vi "Read Write Tests.vi"() -> ()   [LabVIEW 2021]
uses:
  <vilib>/Utility/Data Type/Type Definitions/Data Type.ctl
  <vilib>/TSA/Abstract Data Classes/Abs_Types/Type/Abs_Type.lvclass/Abs_Type.ctl
  Source/Omni-Bus/Omni_Bus.lvclass/Omni_Bus.ctl
  <vilib>/numeric/Random Number (Range) DBL.vi
  <vilib>/numeric/Random Number (Range) U64.vi
  <vilib>/numeric/Random Number (Range) I64.vi
  06a09804-3647-462b-9f8c-3b197f1d4842.vi
  d9e1931d-83c0-4008-a806-d0619767ccd4.vi
  22e3d29d-9de6-4bed-be07-da4388afe74d.vi
  4d5f569c-3ff8-4da6-911e-f6f6b6df5b4c.vi
  853aedcb-843d-4c1a-a070-a8abb42bd888.vi
  632325dd-8024-4226-85a2-78607102a822.vi
  31fcc082-04f4-426e-a822-d083f26efec9.vi
  a6d8fe4b-b8f8-4192-bfbd-ab0450d87a95.vi
  60e7b694-5e2b-40ae-be6d-936c5daed67f.vi
  0a5da363-2ab2-4b0a-bc23-95381a2f4f1f.vi
  f176570a-d467-4534-a5f4-80a5ed2f55fd.vi
  42086b41-aaa2-440a-9863-075bc68471ca.vi
  d6543037-67c4-4c9e-be04-516eba5ce324.vi
  8ee9f7fe-6a64-49fa-a0e4-dd7eef8eba2e.vi
  c8d26da6-dc4a-4689-8e38-86b886253208.vi
  282c234f-af01-4377-8eb2-d0f7920fef08.vi
  a689f72a-6438-4197-ae87-f9cf3b6f7a86.vi
  09187ef5-af96-4de4-9c12-a857a6033bec.vi
  d925c075-5a4f-45eb-b126-c84cbd9bef73.vi
  dbdc5551-9942-400f-9b9d-33a0d6ab74db.vi
  08a2d3fc-7221-4f6a-b613-8a00cd6bc1d4.vi
  211b282e-f175-4618-a45f-9254b3ae1368.vi
  ca77a7b4-ad37-4b73-9f94-404432450396.vi
  2a4b2bb2-c1db-44be-aa83-23dddfec57d5.vi
  b3c2ed11-8a20-4c33-b4f9-0e339c2323c2.vi
  ea50ac27-ce8e-4503-a9f0-9b9e5a91e659.vi
  6f7ce29f-c036-4842-ab22-8910a6a27a54.vi
  616da66d-3857-44c4-988f-95ea5e7f4ed6.vi
  b019b59e-0990-4c2e-a256-e10801dc45bc.vi
  c5feee88-916b-4341-8605-21dc42a231f5.vi
  3d3526cb-8a6e-48a6-bcab-e135716888a1.vi
  6cad3b51-a010-41ec-acd3-d4bb5fa17f8d.vi
  d0c0237e-e14a-450b-9942-79ec582db24b.vi
  ed5cb6ea-b411-43ee-bff1-ba243916202c.vi
  3a337c37-9261-480e-ae0e-8ba3684aa683.vi
  31c5e605-baef-4711-a879-1a5cd8a7ece4.vi
  4ecc3a5c-e12d-463c-8205-51799ca70095.vi
  330bfda6-5fcb-417b-a1fa-665fbbeb5077.vi
  9bcd3a16-7285-4366-9dfb-d430f520f572.vi
  <vilib>/numeric/sub_Random U32.vi
  Source/Omni-Bus/Write.vi
  Source/Omni-Bus/Support/Write/Write SGL.vi
  Source/Omni-Bus/Read.vi
  Source/Omni-Bus/Support/Read/Read SGL.vi
  Source/Omni-Bus/Support/Write/Write DBL.vi
  Source/Omni-Bus/Support/Read/Read DBL.vi
  Source/Omni-Bus/Support/Write/Write EXT.vi
  Source/Omni-Bus/Support/Read/Read EXT.vi
  Source/Omni-Bus/Support/Write/Write CSGL.vi
  Source/Omni-Bus/Support/Read/Read CSGL.vi
  Source/Omni-Bus/Support/Write/Write CDBL.vi
  Source/Omni-Bus/Support/Read/Read CDBL.vi
  Source/Omni-Bus/Support/Write/Write CEXT.vi
  Source/Omni-Bus/Support/Read/Read CEXT.vi
  Source/Omni-Bus/Support/Write/Write I8.vi
  Source/Omni-Bus/Support/Read/Read I8.vi
  Source/Omni-Bus/Support/Write/Write I16.vi
  Source/Omni-Bus/Support/Read/Read I16.vi
  Source/Omni-Bus/Support/Write/Write I32.vi
  Source/Omni-Bus/Support/Read/Read I32.vi
  Source/Omni-Bus/Support/Write/Write I64.vi
  Source/Omni-Bus/Support/Read/Read I64.vi
  Source/Omni-Bus/Support/Write/Write U8.vi
  Source/Omni-Bus/Support/Read/Read U8.vi
  Source/Omni-Bus/Support/Write/Write U16.vi
  Source/Omni-Bus/Support/Read/Read U16.vi
  Source/Omni-Bus/Support/Write/Write U32.vi
  Source/Omni-Bus/Support/Read/Read U32.vi
  Source/Omni-Bus/Support/Write/Write U64.vi
  Source/Omni-Bus/Support/Read/Read U64.vi
  Source/Omni-Bus/Support/Write/Write Time.vi
  Source/Omni-Bus/Support/Read/Read Time.vi
  Source/Omni-Bus/Support/Write/Write Boolean.vi
  Source/Omni-Bus/Support/Read/Read Boolean.vi
  Source/Omni-Bus/Support/Write/Write String.vi
  Source/Omni-Bus/Support/Read/Read String.vi
  Source/Omni-Bus/Support/Write/Write Variant.vi
  Source/Omni-Bus/Support/Read/Read Variant.vi
  Source/Omni-Bus/Support/Write/Write Waveform.vi
  Source/Omni-Bus/Support/Read/Read Waveform.vi
  Source/Omni-Bus/Support/Write/Write Multi SGL.vi
  Source/Omni-Bus/Support/Read/Read Multi SGL.vi
  Source/Omni-Bus/Support/Write/Write Multi DBL.vi
  Source/Omni-Bus/Support/Read/Read Multi DBL.vi
  Source/Omni-Bus/Support/Write/Write Multi EXT.vi
  Source/Omni-Bus/Support/Read/Read Multi EXT.vi
  Source/Omni-Bus/Support/Write/Write Multi CSGL.vi
  Source/Omni-Bus/Support/Read/Read Multi CSGL.vi
  Source/Omni-Bus/Support/Write/Write Multi CDBL.vi
  Source/Omni-Bus/Support/Read/Read Multi CDBL.vi
  Source/Omni-Bus/Support/Write/Write Multi CEXT.vi
  Source/Omni-Bus/Support/Read/Read Multi CEXT.vi
  Source/Omni-Bus/Support/Write/Write Multi I8.vi
  Source/Omni-Bus/Support/Read/Read Multi I8.vi
  Source/Omni-Bus/Support/Write/Write Multi I16.vi
  Source/Omni-Bus/Support/Read/Read Multi I16.vi
  Source/Omni-Bus/Support/Write/Write Multi I32.vi
  Source/Omni-Bus/Support/Read/Read Multi I32.vi
  Source/Omni-Bus/Support/Write/Write Multi I64.vi
  Source/Omni-Bus/Support/Read/Read Multi I64.vi
  Source/Omni-Bus/Support/Write/Write Multi U8.vi
  Source/Omni-Bus/Support/Read/Read Multi U8.vi
  Source/Omni-Bus/Support/Write/Write Multi U16.vi
  Source/Omni-Bus/Support/Read/Read Multi U16.vi
  Source/Omni-Bus/Support/Write/Write Multi U32.vi
  Source/Omni-Bus/Support/Read/Read Multi U32.vi
  Source/Omni-Bus/Support/Write/Write Multi U64.vi
  Source/Omni-Bus/Support/Read/Read Multi U64.vi
  Source/Omni-Bus/Support/Write/Write Multi Time.vi
  Source/Omni-Bus/Support/Read/Read Multi Time.vi
  Source/Omni-Bus/Support/Write/Write Multi Boolean.vi
  Source/Omni-Bus/Support/Read/Read Multi Boolean.vi
  Source/Omni-Bus/Support/Write/Write Multi String.vi
  Source/Omni-Bus/Support/Read/Read Multi String.vi
  Source/Omni-Bus/Support/Write/Write Multi Variant.vi
  Source/Omni-Bus/Support/Read/Read Multi Variant.vi
  Source/Omni-Bus/Support/Write/Write Multi Waveform.vi
  Source/Omni-Bus/Support/Read/Read Multi Waveform.vi
  Source/Omni-Bus/Support/FindVar.vi
  Source/Omni-Bus/Support/Get/Get Multi SGL.vi
  Source/Omni-Bus/Support/Get/Get Multi DBL.vi
  Source/Omni-Bus/Support/Get/Get Multi EXT.vi
  Source/Omni-Bus/Support/Get/Get Multi CPLX_SGL.vi
  Source/Omni-Bus/Support/Get/Get Multi CPLX_DBL.vi
  Source/Omni-Bus/Support/Get/Get Multi CPLX_EXT.vi
  Source/Omni-Bus/Support/Get/Get Multi I8.vi
  Source/Omni-Bus/Support/Get/Get Multi I16.vi
  Source/Omni-Bus/Support/Get/Get Multi I32.vi
  Source/Omni-Bus/Support/Get/Get Multi I64.vi
  Source/Omni-Bus/Support/Get/Get Multi U8.vi
  Source/Omni-Bus/Support/Get/Get Multi U16.vi
  Source/Omni-Bus/Support/Get/Get Multi U32.vi
  Source/Omni-Bus/Support/Get/Get Multi U64.vi
  Source/Omni-Bus/Support/Get/Get Multi Time.vi
  Source/Omni-Bus/Support/Get/Get Multi Boolean.vi
  Source/Omni-Bus/Support/Get/Get Multi String.vi
  Source/Omni-Bus/Support/Get/Get Multi Variant.vi
  Source/Omni-Bus/Support/Get/Get Multi Waveform.vi
  <vilib>/Utility/error.llb/Clear Errors.vi
  Source/Omni-Bus/Properties/Read Var Map.vi
  <vilib>/TSA/Abstract Data Classes/Abs_Types/Type/Properties/Read Tag.vi
  Source/Omni-Bus/Support/FindMultiVar.vi
  Source/Local Bus/Local Bus.lvclass
  C:/Users/Tim/Documents/GitHub/Omni-Bus/Source/Omni-Bus/Bus Access/Bus_Access.lvclass
  <vilib>/TSA/Abstract Data Classes/Abs_Types/Single Float/Abs_Single Float.lvclass
  C:/Program Files (x86)/National Instruments/LabVIEW 2021/vi.lib/TSA/Abstract Data Classes/Abs_Types/Type/Abs_Type.lvclass
  <vilib>/TSA/Abstract Data Classes/Abs_Types/Value/Abs_Value.lvclass
  <vilib>/TSA/Abstract Data Classes/Abs_Types/Double Float/Abs_Double Float.lvclass
  <vilib>/TSA/Abstract Data Classes/Abs_Types/Extended Float/Abs_Extended Float.lvclass
  <vilib>/TSA/Abstract Data Classes/Abs_Types/Complex Single Float/Abs_Complex Single Float.lvclass
  <vilib>/TSA/Abstract Data Classes/Abs_Types/Complex Double Float/Abs_Complex Double Float.lvclass
  <vilib>/TSA/Abstract Data Classes/Abs_Types/Complex Extended Float/Abs_Complex Extended Float.lvclass
  <vilib>/TSA/Abstract Data Classes/Abs_Types/I8 Integer/Abs_I8 Integer.lvclass
  <vilib>/TSA/Abstract Data Classes/Abs_Types/I16 Integer/Abs_I16 Integer.lvclass
  <vilib>/TSA/Abstract Data Classes/Abs_Types/I32 Integer/Abs_I32 Integer.lvclass
  <vilib>/TSA/Abstract Data Classes/Abs_Types/I64 Integer/Abs_I64 Integer.lvclass
  <vilib>/TSA/Abstract Data Classes/Abs_Types/U8 Integer/Abs_U8 Integer.lvclass
  <vilib>/TSA/Abstract Data Classes/Abs_Types/U16 Integer/Abs_U16 Integer.lvclass
  <vilib>/TSA/Abstract Data Classes/Abs_Types/U32 Integer/Abs_U32 Integer.lvclass
  <vilib>/TSA/Abstract Data Classes/Abs_Types/U64 Integer/Abs_U64 Integer.lvclass
  <vilib>/TSA/Abstract Data Classes/Abs_Types/Time/Abs_Time.lvclass
  <vilib>/TSA/Abstract Data Classes/Abs_Types/Boolean/Abs_Boolean.lvclass
  <vilib>/TSA/Abstract Data Classes/Abs_Types/String/Abs_String.lvclass
  <vilib>/TSA/Abstract Data Classes/Abs_Types/Variant/Abs_Variant.lvclass
  <vilib>/TSA/Abstract Data Classes/Abs_Types/Waveform/Abs_Waveform.lvclass
  <vilib>/addons/_JKI Toolkits/Caraya/classes/Test/Define Test.vi
  Source/Local Bus/Initialise - From List.vi
  Source/Omni-Bus/Support/Check For Read Only Error.vi
  Source/Omni-Bus/Support/Incorrect Tag String Error.vi
  <vilib>/addons/_JKI Toolkits/Caraya/classes/Assert/Assert.vi
  <vilib>/addons/_JKI Toolkits/Caraya/classes/Assert/Assert Not Error.vi
  <vilib>/addons/_JKI Toolkits/Caraya/classes/Assert/Assert Equal Value_Variant.vi
  Source/Omni-Bus/Omni_Bus.lvclass
  <vilib>/TSA/Abstract Data Classes/Abs_Types/Type/Abs_Type.lvclass
  <vilib>/Utility/Data Type/NI_Data Type.lvlib
  <vilib>/measure/NI_MAPro.lvlib
  <vilib>/measure/NI_MABase.lvlib
panel:
  out "error out":errorcluster
  in  "error in (no error)":errorcluster
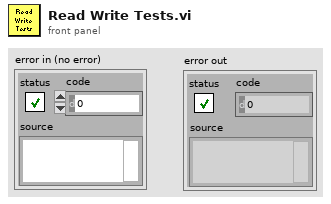
[diagram p1: front panel]
types:
  T1 = typedef "NI_Data Type.lvlib/Data Type.ctl" = enum8{"Invalid Type", "Void", "I8", "I16", "I32", "I64", "U8", "U16", "U32", "U64", "Single Float", "Double Float", "Extended Float", "Single Complex", "Double Complex", "Extended Complex", "Enum U8", "Enum U16", "Enum U32", "Enum U64", "Single Float With Unit", "Double Float With Unit", "Extended Float With Unit", "Single Complex with Unit", "Double Complex with Unit", "Extended Complex with Unit", "Boolean", "String", "Path", "Picture", "Tag", "Array", "Cluster", "Variant", "LV Variant", "Waveform", "Timestamp", "Digital Waveform", "Digital Data", "ExpressData", "Refnum", "External Data", "VI", "Poly VI", "LabVIEW Class Instance", "Fixed Point", "Set Collection", "Map Collection"}
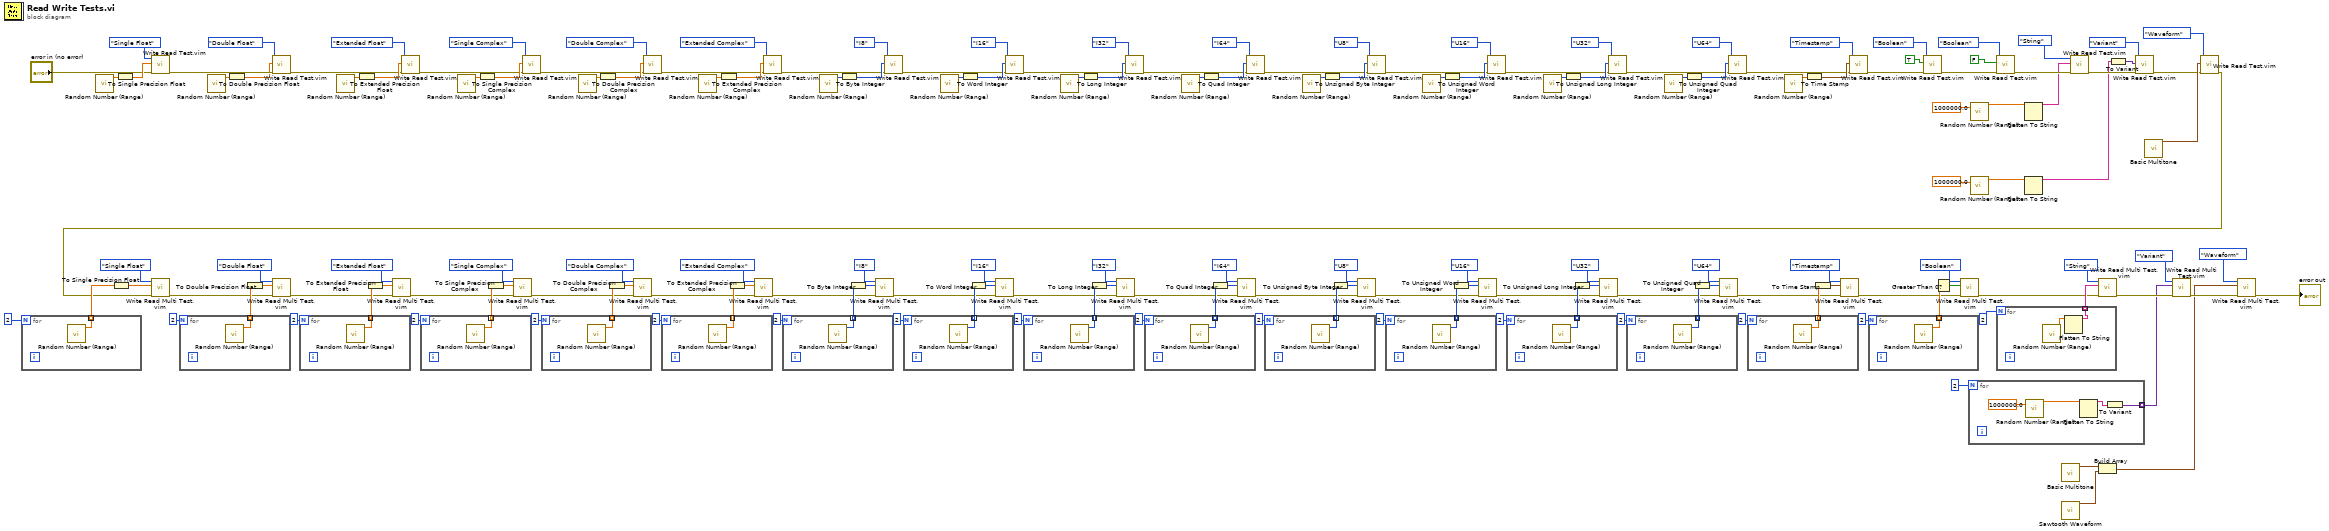
[diagram p0: block diagram]
diagram:
  n1 = for {
    N: 2 -> [_]
    tunnel: [w175] -> w92 mode=indexing
    n2 = call-poly <vilib>:"Random Number (Range).vi"() -> ("number"=w175:dbl)  [unwired: 11 in]
  }
  n3 = call-poly <vilib>:"Random Number (Range).vi"() -> ("number"=w171:dbl)  [unwired: 11 in]
  n4 = To Single Precision Float(number=w92) -> (single precision float=w91:sgl[])
  n5 = To Single Precision Float(number=w171) -> (single precision float=w170:sgl)
  n6 = call "Write Read Test.vim"("error in (no error)"="error in (no error)", "Test Value"=w170, "Type"=Data_Type."Single Float") -> ("error out"=w173:errorcluster)  [unwired: 8 in]
  n7 = for {
    N: 2 -> [_]
    tunnel: [w176] -> w88 mode=indexing
    n8 = call-poly <vilib>:"Random Number (Range).vi"() -> ("number"=w176:dbl)  [unwired: 11 in]
  }
  n9 = call-poly <vilib>:"Random Number (Range).vi"() -> ("number"=w169:dbl)  [unwired: 11 in]
  n10 = To Double Precision Float(number=w169) -> (double precision float=w168:dbl)
  n11 = To Double Precision Float(number=w88) -> (double precision float=w89:dbl[])
  n12 = call "Write Read Test.vim"("error in (no error)"=w173, "Test Value"=w168, "Type"=Data_Type."Double Float") -> ("error out"=w164:errorcluster)  [unwired: 8 in]
  n13 = for {
    N: 2 -> [_]
    tunnel: [w177] -> w82 mode=indexing
    n14 = call-poly <vilib>:"Random Number (Range).vi"() -> ("number"=w177:dbl)  [unwired: 11 in]
  }
  n15 = call-poly <vilib>:"Random Number (Range).vi"() -> ("number"=w166:dbl)  [unwired: 11 in]
  n16 = To Extended Precision Float(1:w166) -> (0:w167:ext)
  n17 = To Extended Precision Float(1:w82) -> (0:w81:ext[])
  n18 = call "Write Read Test.vim"("error in (no error)"=w164, "Test Value"=w167, "Type"=Data_Type."Extended Float") -> ("error out"=w160:errorcluster)  [unwired: 8 in]
  n19 = for {
    N: 2 -> [_]
    tunnel: [w178] -> w79 mode=indexing
    n20 = call-poly <vilib>:"Random Number (Range).vi"() -> ("number"=w178:dbl)  [unwired: 11 in]
  }
  n21 = call-poly <vilib>:"Random Number (Range).vi"() -> ("number"=w162:dbl)  [unwired: 11 in]
  n22 = To Single Precision Complex(1:w162) -> (0:w161:csg)
  n23 = To Single Precision Complex(1:w79) -> (0:w80:csg[])
  n24 = call "Write Read Test.vim"("error in (no error)"=w160, "Test Value"=w161, "Type"=Data_Type."Single Complex") -> ("error out"=w156:errorcluster)  [unwired: 8 in]
  n25 = for {
    N: 2 -> [_]
    tunnel: [w179] -> w74 mode=indexing
    n26 = call-poly <vilib>:"Random Number (Range).vi"() -> ("number"=w179:dbl)  [unwired: 11 in]
  }
  n27 = call-poly <vilib>:"Random Number (Range).vi"() -> ("number"=w158:dbl)  [unwired: 11 in]
  n28 = To Double Precision Complex(1:w158) -> (0:w159:cdb)
  n29 = To Double Precision Complex(1:w74) -> (0:w73:cdb[])
  n30 = call "Write Read Test.vim"("error in (no error)"=w156, "Test Value"=w159, "Type"=Data_Type."Double Complex") -> ("error out"=w152:errorcluster)  [unwired: 8 in]
  n31 = for {
    N: 2 -> [_]
    tunnel: [w180] -> w71 mode=indexing
    n32 = call-poly <vilib>:"Random Number (Range).vi"() -> ("number"=w180:dbl)  [unwired: 11 in]
  }
  n33 = call-poly <vilib>:"Random Number (Range).vi"() -> ("number"=w154:dbl)  [unwired: 11 in]
  n34 = To Extended Precision Complex(1:w154) -> (0:w153:cxt)
  n35 = To Extended Precision Complex(1:w71) -> (0:w72:cxt[])
  n36 = call "Write Read Test.vim"("error in (no error)"=w152, "Test Value"=w153, "Type"=Data_Type."Extended Complex") -> ("error out"=w148:errorcluster)  [unwired: 8 in]
  n37 = for {
    N: 2 -> [_]
    tunnel: [w181] -> w66 mode=indexing
    n38 = call-poly <vilib>:"Random Number (Range).vi"() -> ("number"=w181:i64)  [unwired: 11 in]
  }
  n39 = call-poly <vilib>:"Random Number (Range).vi"() -> ("number"=w150:i64)  [unwired: 11 in]
  n40 = To Byte Integer(number=w150) -> (8bit integer=w151:i8)
  n41 = To Byte Integer(number=w66) -> (8bit integer=w65:i8[])
  n42 = call "Write Read Test.vim"("error in (no error)"=w148, "Test Value"=w151, "Type"=Data_Type."I8") -> ("error out"=w144:errorcluster)  [unwired: 8 in]
  n43 = for {
    N: 2 -> [_]
    tunnel: [w182] -> w63 mode=indexing
    n44 = call-poly <vilib>:"Random Number (Range).vi"() -> ("number"=w182:i64)  [unwired: 11 in]
  }
  n45 = call-poly <vilib>:"Random Number (Range).vi"() -> ("number"=w146:i64)  [unwired: 11 in]
  n46 = To Word Integer(number=w146) -> (16bit integer=w145:i16)
  n47 = To Word Integer(number=w63) -> (16bit integer=w64:i16[])
  n48 = call "Write Read Test.vim"("error in (no error)"=w144, "Test Value"=w145, "Type"=Data_Type."I16") -> ("error out"=w140:errorcluster)  [unwired: 8 in]
  n49 = for {
    N: 2 -> [_]
    tunnel: [w183] -> w58 mode=indexing
    n50 = call-poly <vilib>:"Random Number (Range).vi"() -> ("number"=w183:i64)  [unwired: 11 in]
  }
  n51 = call-poly <vilib>:"Random Number (Range).vi"() -> ("number"=w142:i64)  [unwired: 11 in]
  n52 = To Long Integer(number=w142) -> (32bit integer=w143:i32)
  n53 = To Long Integer(number=w58) -> (32bit integer=w57:i32[])
  n54 = call "Write Read Test.vim"("error in (no error)"=w140, "Test Value"=w143, "Type"=Data_Type."I32") -> ("error out"=w136:errorcluster)  [unwired: 8 in]
  n55 = for {
    N: 2 -> [_]
    tunnel: [w184] -> w55 mode=indexing
    n56 = call-poly <vilib>:"Random Number (Range).vi"() -> ("number"=w184:i64)  [unwired: 11 in]
  }
  n57 = call-poly <vilib>:"Random Number (Range).vi"() -> ("number"=w138:i64)  [unwired: 11 in]
  n58 = To Quad Integer(1:w138) -> (0:w137:i64)
  n59 = To Quad Integer(1:w55) -> (0:w56:i64[])
  n60 = call "Write Read Test.vim"("error in (no error)"=w136, "Test Value"=w137, "Type"=Data_Type."I64") -> ("error out"=w132:errorcluster)  [unwired: 8 in]
  n61 = for {
    N: 2 -> [_]
    tunnel: [w185] -> w50 mode=indexing
    n62 = call-poly <vilib>:"Random Number (Range).vi"() -> ("number"=w185:u64)  [unwired: 11 in]
  }
  n63 = call-poly <vilib>:"Random Number (Range).vi"() -> ("number"=w134:u64)  [unwired: 11 in]
  n64 = To Unsigned Byte Integer(number=w134) -> (unsigned 8bit integer=w135:u8)
  n65 = To Unsigned Byte Integer(number=w50) -> (unsigned 8bit integer=w49:u8[])
  n66 = call "Write Read Test.vim"("error in (no error)"=w132, "Test Value"=w135, "Type"=Data_Type."U8") -> ("error out"=w128:errorcluster)  [unwired: 8 in]
  n67 = for {
    N: 2 -> [_]
    tunnel: [w186] -> w47 mode=indexing
    n68 = call-poly <vilib>:"Random Number (Range).vi"() -> ("number"=w186:u64)  [unwired: 11 in]
  }
  n69 = call-poly <vilib>:"Random Number (Range).vi"() -> ("number"=w130:u64)  [unwired: 11 in]
  n70 = To Unsigned Word Integer(number=w130) -> (unsigned 16bit integer=w129:u16)
  n71 = To Unsigned Word Integer(number=w47) -> (unsigned 16bit integer=w48:u16[])
  n72 = call "Write Read Test.vim"("error in (no error)"=w128, "Test Value"=w129, "Type"=Data_Type."U16") -> ("error out"=w124:errorcluster)  [unwired: 8 in]
  n73 = for {
    N: 2 -> [_]
    tunnel: [w187] -> w42 mode=indexing
    n74 = call-poly <vilib>:"Random Number (Range).vi"() -> ("number"=w187:u64)  [unwired: 11 in]
  }
  n75 = call-poly <vilib>:"Random Number (Range).vi"() -> ("number"=w126:u64)  [unwired: 11 in]
  n76 = To Unsigned Long Integer(number=w126) -> (unsigned 32bit integer=w127:u32)
  n77 = To Unsigned Long Integer(number=w42) -> (unsigned 32bit integer=w41:u32[])
  n78 = call "Write Read Test.vim"("error in (no error)"=w124, "Test Value"=w127, "Type"=Data_Type."U32") -> ("error out"=w120:errorcluster)  [unwired: 8 in]
  n79 = for {
    N: 2 -> [_]
    tunnel: [w188] -> w39 mode=indexing
    n80 = call-poly <vilib>:"Random Number (Range).vi"() -> ("number"=w188:u64)  [unwired: 11 in]
  }
  n81 = call-poly <vilib>:"Random Number (Range).vi"() -> ("number"=w122:u64)  [unwired: 11 in]
  n82 = To Unsigned Quad Integer(1:w122) -> (0:w121:u64)
  n83 = To Unsigned Quad Integer(1:w39) -> (0:w40:u64[])
  n84 = call "Write Read Test.vim"("error in (no error)"=w120, "Test Value"=w121, "Type"=Data_Type."U64") -> ("error out"=w115:errorcluster)  [unwired: 8 in]
  n85 = for {
    N: 2 -> [_]
    tunnel: [w189] -> w34 mode=indexing
    n86 = call-poly <vilib>:"Random Number (Range).vi"() -> ("number"=w189:dbl)  [unwired: 11 in]
  }
  n87 = call-poly <vilib>:"Random Number (Range).vi"() -> ("number"=w117:dbl)  [unwired: 11 in]
  n88 = To Time Stamp(1:w117) -> (0:w118:timestamp)
  n89 = To Time Stamp(1:w34) -> (0:w33:timestamp[])
  n90 = call "Write Read Test.vim"("error in (no error)"=w115, "Test Value"=w118, "Type"=Data_Type."Timestamp") -> ("error out"=w112:errorcluster)  [unwired: 8 in]
  n91 = for {
    N: 2 -> [_]
    tunnel: [w190] -> w31 mode=indexing
    n92 = call-poly <vilib>:"Random Number (Range).vi"() -> ("number"=w190:dbl)  [unwired: 11 in]
  }
  n93 = call "Write Read Test.vim"("error in (no error)"=w112, "Test Value"=TRUE, "Type"=Data_Type."Boolean") -> ("error out"=w109:errorcluster)  [unwired: 8 in]
  n94 = Greater Than 0?(x=w31) -> (x > 0?=w32:bool[])
  n95 = for {
    N: 2 -> [_]
    tunnel: [w191] -> w9 mode=indexing
    n96 = call-poly <vilib>:"Random Number (Range).vi"("upper bound (100)"=1000000.0) -> ("number"=w194:dbl)  [unwired: 10 in]
    n97 = Flatten To String(anything=w194) -> (data string=w192:string)  [unwired: 3 in, 2 out]
    n98 = To Variant(anything=w192) -> (Variant=w191:variant)
  }
  n99 = call-poly <vilib>:"Random Number (Range).vi"("upper bound (100)"=1000000.0) -> ("number"=w104:dbl)  [unwired: 10 in]
  n100 = call-poly <vilib>:"Random Number (Range).vi"("upper bound (100)"=1000000.0) -> ("number"=w99:dbl)  [unwired: 10 in]
  n101 = call "Write Read Test.vim"("error in (no error)"=w109, "Test Value"=FALSE, "Type"=Data_Type."Boolean") -> ("error out"=w106:errorcluster)  [unwired: 8 in]
  n102 = for {
    N: 2 -> [_]
    tunnel: [w196] -> w26 mode=indexing
    n103 = call-poly <vilib>:"Random Number (Range).vi"() -> ("number"=w195:dbl)  [unwired: 11 in]
    n104 = Flatten To String(anything=w195) -> (data string=w196:string)  [unwired: 3 in, 2 out]
  }
  n105 = Flatten To String(anything=w104) -> (data string=w105:string)  [unwired: 3 in, 2 out]
  n106 = Flatten To String(anything=w99) -> (data string=w98:string)  [unwired: 3 in, 2 out]
  n107 = call <vilib>:"Basic Multitone.vi"() -> ("signal out"=w3:waveform(dbl))  [unwired: 12 in, 3 out]
  n108 = call <vilib>:"Sawtooth Waveform.vi"() -> ("signal out"=w1:waveform(dbl))  [unwired: 10 in, 1 out]
  n109 = call "Write Read Test.vim"("error in (no error)"=w106, "Test Value"=w105, "Type"=Data_Type."String") -> ("error out"=w102:errorcluster)  [unwired: 8 in]
  n110 = Build Array(w3, w1) -> (w2:waveform(dbl)[])
  n111 = To Variant(anything=w98) -> (Variant=w101:variant)
  n112 = call "Write Read Test.vim"("error in (no error)"=w102, "Test Value"=w101, "Type"=Data_Type."Variant") -> ("error out"=w95:errorcluster)  [unwired: 8 in]
  n113 = call <vilib>:"Basic Multitone.vi"() -> ("signal out"=w96:waveform(dbl))  [unwired: 12 in, 3 out]
  n114 = call "Write Read Test.vim"("error in (no error)"=w95, "Test Value"=w96, "Type"=Data_Type."Waveform") -> ("error out"=w90:errorcluster)  [unwired: 8 in]
  n115 = call "Write Read Multi Test.vim"("error in (no error)"=w90, "Test Value"=w91, "Type"=Data_Type."Single Float") -> ("error out"=w85:errorcluster)  [unwired: 8 in]
  n116 = call "Write Read Multi Test.vim"("error in (no error)"=w85, "Test Value"=w89, "Type"=Data_Type."Double Float") -> ("error out"=w25:errorcluster)  [unwired: 8 in]
  n117 = call "Write Read Multi Test.vim"("error in (no error)"=w25, "Test Value"=w81, "Type"=Data_Type."Extended Float") -> ("error out"=w24:errorcluster)  [unwired: 8 in]
  n118 = call "Write Read Multi Test.vim"("error in (no error)"=w24, "Test Value"=w80, "Type"=Data_Type."Single Complex") -> ("error out"=w23:errorcluster)  [unwired: 8 in]
  n119 = call "Write Read Multi Test.vim"("error in (no error)"=w23, "Test Value"=w73, "Type"=Data_Type."Double Complex") -> ("error out"=w22:errorcluster)  [unwired: 8 in]
  n120 = call "Write Read Multi Test.vim"("error in (no error)"=w22, "Test Value"=w72, "Type"=Data_Type."Extended Complex") -> ("error out"=w21:errorcluster)  [unwired: 8 in]
  n121 = call "Write Read Multi Test.vim"("error in (no error)"=w21, "Test Value"=w65, "Type"=Data_Type."I8") -> ("error out"=w20:errorcluster)  [unwired: 8 in]
  n122 = call "Write Read Multi Test.vim"("error in (no error)"=w20, "Test Value"=w64, "Type"=Data_Type."I16") -> ("error out"=w19:errorcluster)  [unwired: 8 in]
  n123 = call "Write Read Multi Test.vim"("error in (no error)"=w19, "Test Value"=w57, "Type"=Data_Type."I32") -> ("error out"=w18:errorcluster)  [unwired: 8 in]
  n124 = call "Write Read Multi Test.vim"("error in (no error)"=w18, "Test Value"=w56, "Type"=Data_Type."I64") -> ("error out"=w17:errorcluster)  [unwired: 8 in]
  n125 = call "Write Read Multi Test.vim"("error in (no error)"=w17, "Test Value"=w49, "Type"=Data_Type."U8") -> ("error out"=w16:errorcluster)  [unwired: 8 in]
  n126 = call "Write Read Multi Test.vim"("error in (no error)"=w16, "Test Value"=w48, "Type"=Data_Type."U16") -> ("error out"=w15:errorcluster)  [unwired: 8 in]
  n127 = call "Write Read Multi Test.vim"("error in (no error)"=w15, "Test Value"=w41, "Type"=Data_Type."U32") -> ("error out"=w14:errorcluster)  [unwired: 8 in]
  n128 = call "Write Read Multi Test.vim"("error in (no error)"=w14, "Test Value"=w40, "Type"=Data_Type."U64") -> ("error out"=w13:errorcluster)  [unwired: 8 in]
  n129 = call "Write Read Multi Test.vim"("error in (no error)"=w13, "Test Value"=w33, "Type"=Data_Type."Timestamp") -> ("error out"=w12:errorcluster)  [unwired: 8 in]
  n130 = call "Write Read Multi Test.vim"("error in (no error)"=w12, "Test Value"=w32, "Type"=Data_Type."Boolean") -> ("error out"=w11:errorcluster)  [unwired: 8 in]
  n131 = call "Write Read Multi Test.vim"("error in (no error)"=w11, "Test Value"=w26, "Type"=Data_Type."String") -> ("error out"=w10:errorcluster)  [unwired: 8 in]
  n132 = call "Write Read Multi Test.vim"("error in (no error)"=w10, "Test Value"=w9, "Type"=Data_Type."Variant") -> ("error out"=w4:errorcluster)  [unwired: 8 in]
  n133 = call "Write Read Multi Test.vim"("error in (no error)"=w4, "Test Value"=w2, "Type"=Data_Type."Waveform") -> ("error out"=→"error out":errorcluster)  [unwired: 8 in]
